vi "Network-Test Discovery Beacon.vi"() -> ()   [LabVIEW 2020]
uses:
  Payloads/Network-Filename Payload.ctl
panel:
  out "Filename":string
  out "command":string
  in  "stop":bool
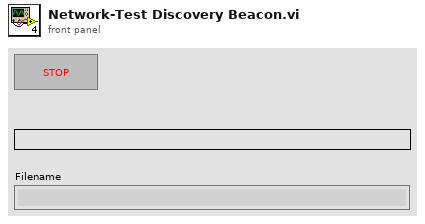
[diagram p1: front panel]
types:
  T1 = typedef "Network-Filename Payload.ctl" = cluster{"Filename":string}
  T2 = typedef "Network-TCP Message.ctl" = cluster{"Code":i32, "Command":string, "Payload":string}
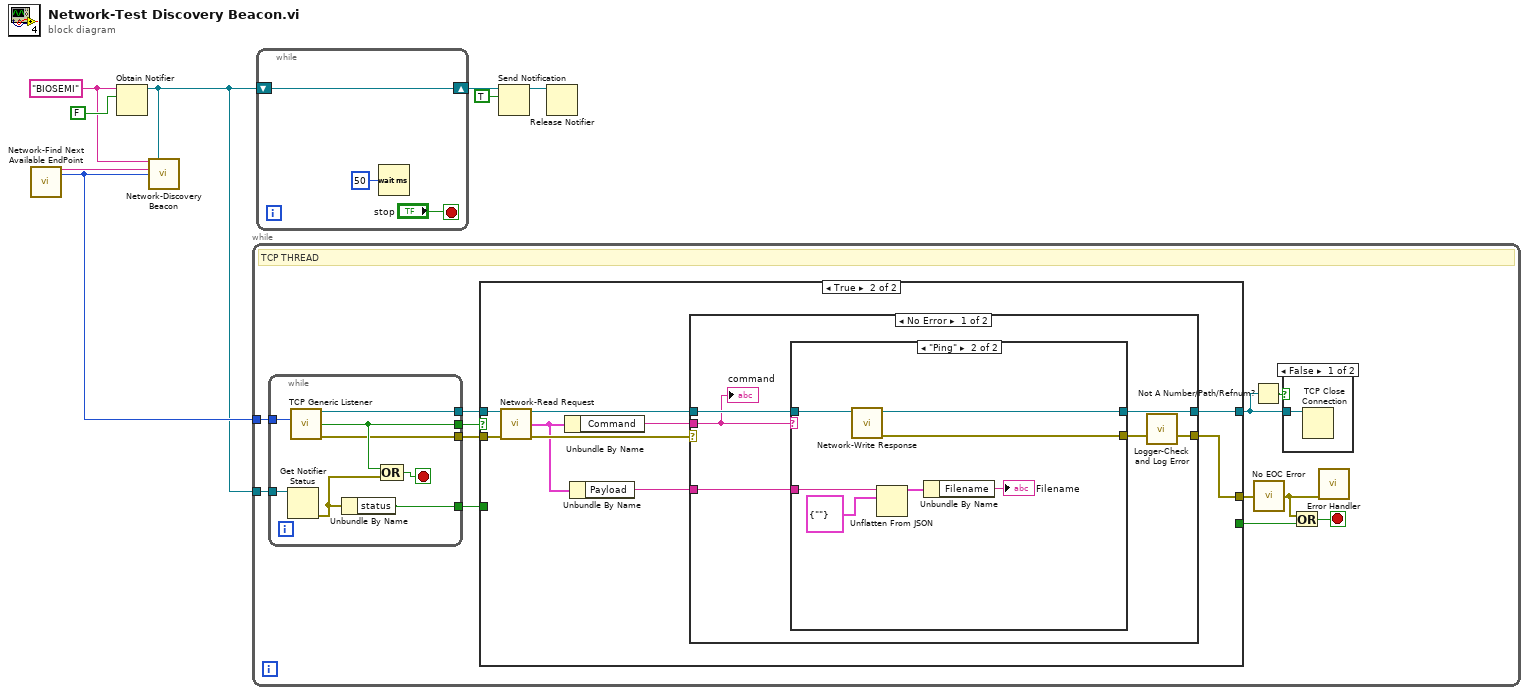
[diagram p0: block diagram]
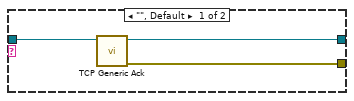
[diagram p3: hidden frame]
diagram:
  w3 = "BIOSEMI" ("name")
  n1 = call "Network-Find Next Available EndPoint.vi"() -> ("address"=w8:string, "port"=w2:u16)  [unwired: 13 in, 1 out]
  n2 = Obtain Notifier(name (unnamed)=w3, notification data type=FALSE) -> (notifier out=w1:refnum<notifier>)  [unwired: 2 in, 2 out]
  n3 = call "Network-Discovery Beacon.vi"("name"=w3, "kill thread notifier"=w1, "tcpAddress"=w8, "tcpPort"=w2) -> ()  [unwired: 12 in]
  n4 = while {
    tunnel: w2 -> [w16]
    tunnel: w1 -> [w11]
    stop <- w12 stop-if-true
    # "TCP THREAD"
    n5 = while {
      tunnel: [w55] -> w20
      tunnel: [w58] -> w19
      tunnel: w16 -> [w56]
      tunnel: [w54] -> w15
      tunnel: w11 -> [w53]
      tunnel: [w51] -> w10
      stop <- w57 stop-if-true
      n6 = Get Notifier Status(notifier=w53) -> (error out=w52:errorcluster)  [unwired: 1 in, 4 out]
      n7 = call "TCP Generic Listener.vi"("port"=w56) -> ("connection ID"=w58:refnum<k5>, "Connected?"=w55:bool, "error out"=w54:errorcluster)  [unwired: 12 in]
      n8 = Unbundle By Name(w52) -> ("status"=w51:bool)
      n9 = Compound Arithmetic op=OR(w55, w52) -> (w57:bool)
    }
    n10 = case shown="True" w20 {
      tunnel: w15 -> [w22 w29]
      tunnel: w19 -> [w23 w30]
      tunnel: [w23 w32] -> w17
      tunnel: [w22 w31] -> w14
      tunnel: w10 -> [w21 _]
      tunnel: [w21 _] -> w9
      frame False {
      }
      frame True {
        n11 = call "Network-Read Request.vi"("connection ID"=w30, "error in (no error)"=w29) -> ("connection ID out"=w28:refnum<k5>, "TCPMessage"=w25:T2, "error out"=w27:errorcluster)  [unwired: 11 in]
        n12 = Unbundle By Name(w25) -> ("Command"=w26:string)
        n13 = Unbundle By Name(w25) -> ("Payload"=w24:string)
        n14 = case shown="No Error" w27 {
          selector: w27 -> [_ w49]
          tunnel: w28 -> [w38 w50]
          tunnel: [w37 w50] -> w32
          tunnel: [w35 w49] -> w31
          tunnel: w26 -> [w34 _]
          tunnel: w24 -> [w33 _]
          frame No Error {
            n15 = case shown="\"Ping\"" w34 {
              tunnel: w38 -> [w41 w48]
              tunnel: [w40 w47] -> w37
              tunnel: [w39 w46] -> w36
              tunnel: w33 -> [_ w45]
              frame "", Default {
                n16 = call "TCP Generic Ack.vi"("connection ID"=w41) -> ("error out"=w39:errorcluster, "connection ID out"=w40:refnum<k5>)  [unwired: 9 in]
              }
              frame "Ping" {
                n17 = call "Network-Write Response.vi"("connection ID"=w48) -> ("connection ID out"=w47:refnum<k5>, "error out"=w46:errorcluster)  [unwired: 13 in]
                n18 = Unflatten From JSON(JSON string=w45, type and defaults=T1 {"Filename"=""} ("FilenamePayload")) -> (value=w43:T1)  [unwired: 5 in, 1 out]
                n19 = Unbundle By Name(w43) -> ("Filename"=→"Filename":string)
              }
            }
            n20 = call "Logger-Check and Log Error.vi"("error in (no error)"=w36) -> ("error out"=w35:errorcluster)  [unwired: 14 in]
            "command" <- w34
          }
          frame Error {
          }
        }
      }
    }
    n21 = Not A Number/Path/Refnum?(number/path/refnum=w17) -> (NaN/Path/Refnum?=w18:bool)
    n22 = call "No EOC Error.vi"("error in"=w14) -> ("error out"=w13:errorcluster)  [unwired: 4 in]
    n23 = case shown="False" w18 {
      tunnel: w17 -> [w59 _]
      frame False {
        n24 = TCP Close Connection(connection ID=w59) -> ()  [unwired: 2 in, 2 out]
      }
      frame True {
      }
    }
    n25 = Or(x=w13, y=w9) -> (x .or. y?=w12:bool)
    n26 = call "Error Handler.vi"("error in (no error)"=w13) -> ()  [unwired: 12 in, 3 out]
  }
  n27 = while {
    shift-right: [w60] -> w6
    shift-left: w1 -> [w60]
    stop <- "stop" stop-if-true
    n28 = Wait (ms)(milliseconds to wait=u32 50) -> ()  [unwired: 1 out]
  }
  n29 = Send Notification(notification=TRUE, notifier=w6) -> (notifier out=w4:refnum<notifier>)  [unwired: 1 in, 1 out]
  n30 = Release Notifier(notifier=w4) -> ()  [unwired: 2 in, 3 out]
